vi "VCS Get Enable State.vi"(8 "error in (no error)":errorcluster, 11 "axis in":cluster{"keyHandle":u32, "nodeId":u16}={"keyHandle"=0, "nodeId"=1}) -> (0 "error out":errorcluster, 2 "isEnabled":i32, 3 "axis out":cluster{"keyHandle":u32, "nodeId":u16}={"keyHandle"=0, "nodeId"=1})   [LabVIEW 2017, in "maxonEPOS.lvlib"]
doc: "<B>VCS Get Enable Stat</B> returns the device state enable (isEnabled = TRUE)."
uses:
  Examples/maxonEPOS.lvlib
  Resources/EposCmd.dll
  SSI_Tool/InstrumentsInterfaces/Motordriver/maxon EPOS/Resources/EposCmd64.dll
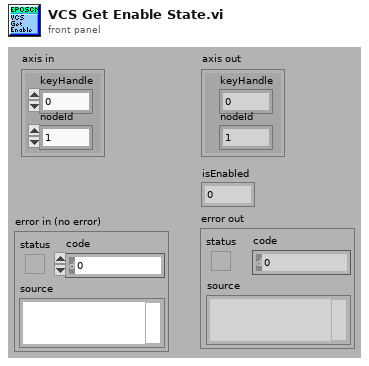
[diagram p1: front panel]
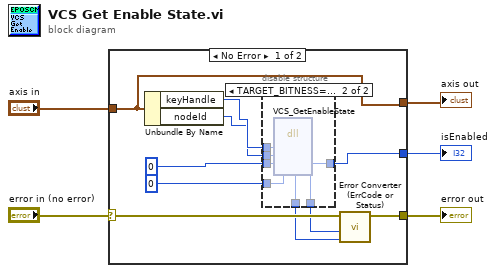
[diagram p0: block diagram]
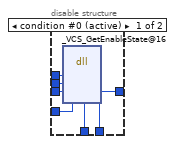
[diagram p2: hidden frame]
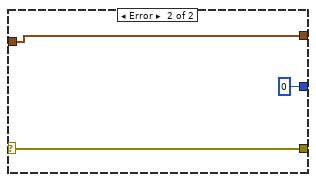
[diagram p3: hidden frame]
diagram:
  n1 = case shown="No Error" "error in (no error)" {
    selector: "error in (no error)" -> [w14 w32]
    tunnel: [w13 w32] -> w4
    tunnel: [w15 0 ("pIsEnabled")] -> w3
    tunnel: "axis in" -> [w6 w31]
    tunnel: [w6 w31] -> w1
    frame No Error {
      n2 = Unbundle By Name(w6) -> ("keyHandle"=w10:u32, "nodeId"=w9:u16)
      n3 = disable-structure shown="TARGET_BITNESS==64" {
        disable-tunnel: [w22 w29] -> w15
        disable-tunnel: [w21 w28] -> w12
        disable-tunnel: [w20 w27] -> w11
        disable-tunnel: w10 -> [w19 w26]
        disable-tunnel: w9 -> [w18 w25]
        disable-tunnel: 0 ("pIsEnabled") -> [w17 w24]
        disable-tunnel: u32 0 ("pErrorCode") -> [w16 w23]
        frame condition #0 (active) {
          n4 = dll-call lib="C:/workspace/project/scancon/sw/SSI_Tool/InstrumentsInterfaces/Motordriver/maxon EPOS/Resources/EposCmd.*" fn="_VCS_GetEnableState@16"("KeyHandle"=w19, "NodeId"=w18, "pIsEnabled"=w17, "pErrorCode"=w16) -> (w21:i32, "pIsEnabled"=w22:i32, "pErrorCode"=w20:u32)  [unwired: 5 in, 2 out]
        }
        frame condition #1 {
          n5 = dll-call lib="C:/Sources/LabView/maxon EPOS/Resources/EposCmd64.*" fn="VCS_GetEnableState" ("EposCmd.dll:_VCS_GetEnableState@16")("KeyHandle"=w26, "NodeId"=w25, "pIsEnabled"=w24, "pErrorCode"=w23) -> ("Rückgabetyp"=w28:i32, "pIsEnabled"=w29:i32, "pErrorCode"=w27:u32)  [unwired: 5 in, 2 out]
        }
      }
      n6 = call "Error Converter (ErrCode or Status).vi"("error code"=w11, "return type"=w12, "error in (no error)"=w14) -> ("error out"=w13:errorcluster)  [unwired: 7 in]
    }
    frame Error {
    }
  }
  "isEnabled" <- w3
  "error out" <- w4
  "axis out" <- w1
